vi "Unit Test.vi"() -> ()   [LabVIEW 2018]
uses:
  Custom Controls/Select Cursor.ctl
  Custom Controls/Analog Channels.ctl
  Custom Controls/Run Control.ctl
  Oscilloscope.lvclass
  Oscilloscope.lvlib
panel:
  in  "Run Control":T1
  in  "Active Channel(s)":T2[](array[typedef])
  out "Waveform":waveform(dbl)(graph)
  in  "Channel":T2
  out "Position":dbl format="%.9f"
  in  "Cursor":T3
  out "Status Array":bool[](array[boolean])
  out "Self-Test Passed?":bool
  out "Cal Passed ? (T:Yes)":bool
  in  "Device":string
  in  "stop":bool
  out "error out":errorcluster
  in  "error in (no error)":errorcluster
  # "---------------------------------------------------------->"
  # "---------------------------------------------------------->"
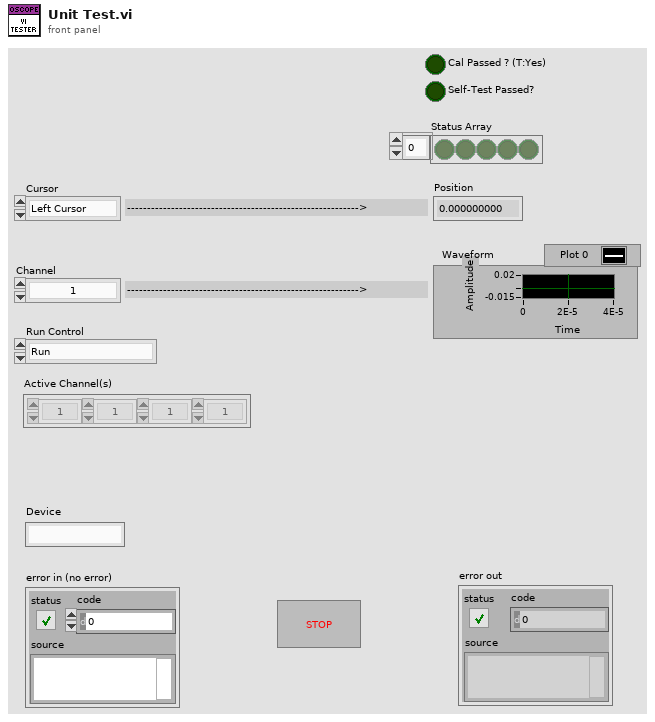
[diagram p1: front panel]
types:
  T1 = typedef "Oscilloscope.lvlib/Run Control.ctl" = enum16{"Run", "Single", "Stop"}
  T2 = typedef "Oscilloscope.lvlib/Analog Channels.ctl" = enum16{"1", "2", "3", "4", "5", "6", "7", "8", "9", "10", "11", "12", "13", "14", "15", "16"}
  T3 = typedef "Oscilloscope.lvlib/Select Cursor.ctl" = enum16{"Left Cursor", "Right Cursor", "Top Cursor", "Bottom Cursor"}
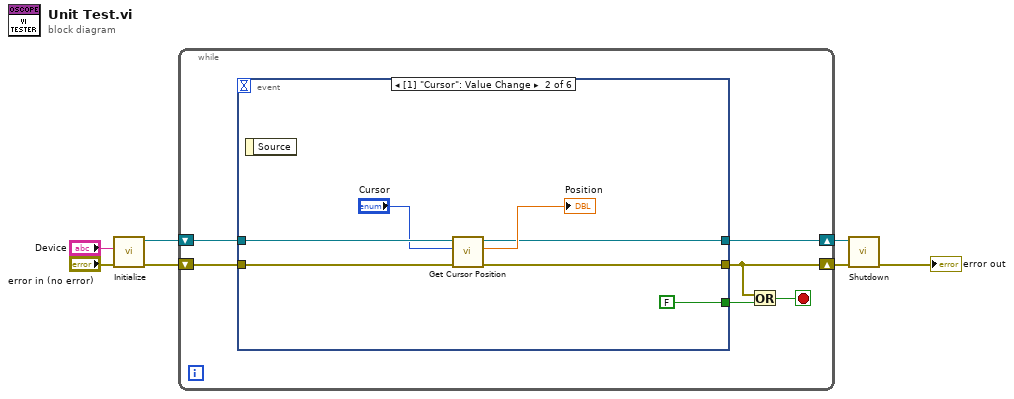
[diagram p0: block diagram]
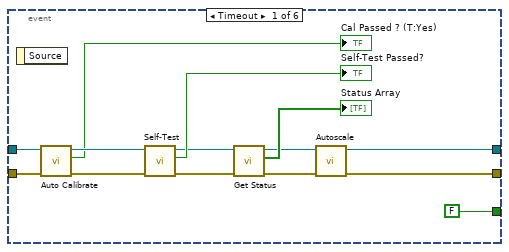
[diagram p2: hidden frame]
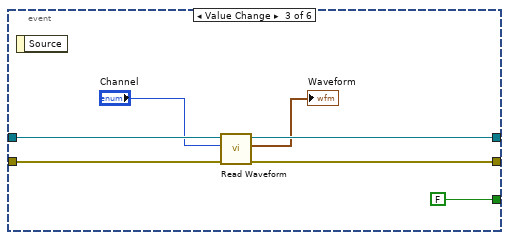
[diagram p3: hidden frame]
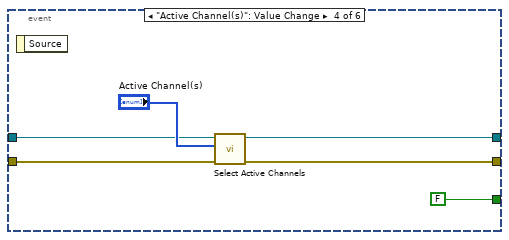
[diagram p4: hidden frame]
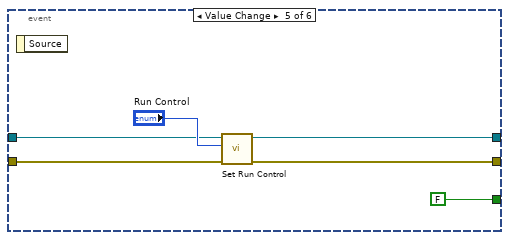
[diagram p5: hidden frame]
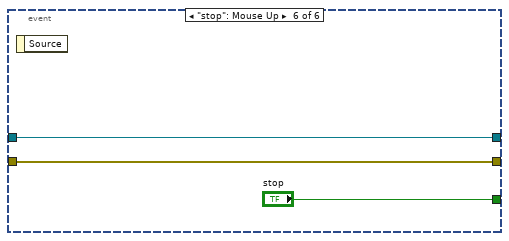
[diagram p6: hidden frame]
diagram:
  n1 = call "Initialize.vi"("error in (no error)"="error in (no error)", "Device"="Device") -> ("error out"=w5:errorcluster, "Oscilloscope"=w7:refnum<class "Oscilloscope.lvclass">)  [unwired: 8 in]
  n2 = while {
    shift-right: [w12] -> w6
    shift-left: w7 -> [w13]
    shift-right: [w10] -> w4
    shift-left: w5 -> [w11]
    stop <- w8 stop-if-true
    n3 = event shown="[1] \"Cursor\": Value Change" {
      selector: _ -> [_ _ _ _ _ _]
      dyn-events: _ -> [_ _ _ _ _ _]
      timeout: _ -> [_ _ _ _ _ _]
      tunnel: [w16 w30 w38 w43 w50 w54] -> w12
      tunnel: w13 -> [w26 w34 w41 w46 w52 w54]
      tunnel: [w14 w29 w37 w44 w49 w56] -> w10
      tunnel: w11 -> [w25 w33 w40 w45 w51 w56]
      tunnel: [FALSE ("stop") FALSE ("stop") FALSE ("stop") FALSE ("stop") FALSE ("stop") "stop"] -> w9
      event Timeout {
        n4 = event-data() -> ()  [unwired: 1 in, 1 out]
        n5 = call-dynamic "Auto Calibrate.vi"("error in (no error)"=w25, "Oscilloscope in"=w26) -> ("error out"=w24:errorcluster, "Cal Passed ? (T:Yes)"=→"Cal Passed ? (T:Yes)":bool, "Oscilloscope out"=w23:refnum<class "Oscilloscope.lvclass">)  [unwired: 7 in]
        n6 = call-dynamic "Self-Test.vi"("error in (no error)"=w24, "Oscilloscope in"=w23) -> ("error out"=w20:errorcluster, "Self-Test Passed? (T:Yes)"=→"Self-Test Passed?":bool, "Oscilloscope out"=w19:refnum<class "Oscilloscope.lvclass">)  [unwired: 7 in]
        n7 = call-dynamic "Get Status.vi"("error in (no error)"=w20, "Oscilloscope in"=w19) -> ("error out"=w15:errorcluster, "Status Array"=→"Status Array":bool[], "Oscilloscope out"=w17:refnum<class "Oscilloscope.lvclass">)  [unwired: 7 in]
        n8 = call-dynamic "Autoscale.vi"("error in (no error)"=w15, "Oscilloscope in"=w17) -> ("error out"=w14:errorcluster, "Oscilloscope out"=w16:refnum<class "Oscilloscope.lvclass">)  [unwired: 8 in]
      }
      event Value Change {
        n9 = event-data() -> ()  [unwired: 1 in, 1 out]
        n10 = call-dynamic "Get Cursor Position.vi"("error in (no error)"=w33, "Cursor"="Cursor", "Oscilloscope in"=w34) -> ("error out"=w29:errorcluster, "Position"=→"Position":dbl, "Oscilloscope out"=w30:refnum<class "Oscilloscope.lvclass">)  [unwired: 6 in]
      }
      event Value Change {
        n11 = event-data() -> ()  [unwired: 1 in, 1 out]
        n12 = call-dynamic "Read Waveform.vi"("error in (no error)"=w40, "Channel"="Channel", "Oscilloscope in"=w41) -> ("error out"=w37:errorcluster, "Waveform"=→"Waveform":waveform(dbl), "Oscilloscope out"=w38:refnum<class "Oscilloscope.lvclass">)  [unwired: 6 in]
      }
      event "Active Channel(s)": Value Change {
        n13 = event-data() -> ()  [unwired: 1 in, 1 out]
        n14 = call-dynamic "Select Active Channels.vi"("error in (no error)"=w45, "Active Channel(s)"="Active Channel(s)", "Oscilloscope in"=w46) -> ("error out"=w44:errorcluster, "Oscilloscope out"=w43:refnum<class "Oscilloscope.lvclass">)  [unwired: 7 in]
      }
      event Value Change {
        n15 = event-data() -> ()  [unwired: 1 in, 1 out]
        n16 = call-dynamic "Set Run Control.vi"("error in (no error)"=w51, "Run Control"="Run Control", "Oscilloscope in"=w52) -> ("error out"=w49:errorcluster, "Oscilloscope out"=w50:refnum<class "Oscilloscope.lvclass">)  [unwired: 7 in]
      }
      event "stop": Mouse Up {
        n17 = event-data() -> ()  [unwired: 1 in, 1 out]
      }
    }
    n18 = Or(x=w10, y=w9) -> (x .or. y?=w8:bool)
  }
  n19 = call "Shutdown.vi"("error in (no error)"=w4, "Oscilloscope in"=w6) -> ("error out"=→"error out":errorcluster)  [unwired: 8 in, 1 out]
